vi "auto_food.vi"(10 "columns":i32[](array[numeric]), 11 "rows":i32[](array[numeric])) -> (3 "angle":dbl)   [LabVIEW 2015, in "PolyVIEW.lvclass"]
uses:
  PolyVIEW.lvclass
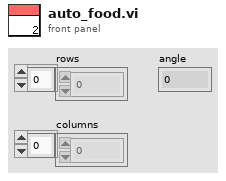
[diagram p1: front panel]
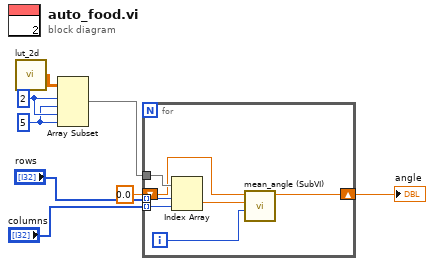
[diagram p0: block diagram]
diagram:
  w6 = 2 ("length")
  w3 = 5 ("length")
  n1 = call "lut_2d.vi"() -> ("output array"=w5:dbl[][])
  n2 = Array Subset(array=w5, index (row)=w6, length (row)=w3, index (col)=w6, length (col)=w3) -> (w4:dbl[][])
  n3 = for {
    tunnel: w4 -> [w15]
    tunnel: "rows" -> [w14] mode=indexing
    tunnel: "columns" -> [w13] mode=indexing
    shift-right: [w11] -> w1
    shift-left: 0.0 ("angle out") -> [w9]
    i -> [w12]
    n4 = Index Array(array=w15, index (row)=w14, index (col)=w13) -> (element=w10:dbl)
    n5 = call "mean_angle (SubVI).vi"("quant"=w12, "angle 2"=w10, "angle 1"=w9) -> ("angle out"=w11:dbl)  [unwired: 8 in]
  }
  "angle" <- w1
